vi "initialize.vi"(8 "error in (no error)":errorcluster, 10 "project_file":path, 11 "lv-builder in":refnum<class "lv-builder-default.lvclass">) -> (0 "error out":errorcluster, 3 "lv-builder out":refnum<class "lv-builder-default.lvclass">)   [LabVIEW 2015, in "lv-builder-default.lvclass"]
uses:
  lv-builder-default.lvclass
  <userlib>/antonio-alexander/lv-bin/lv-bin/public/api/v1/advanced/add_data_path_single.vi
  lv-builder/public/accessors/project_file_write.vi
  lv-builder/public/accessors/commit_hash_write.vi
  lv-builder-default.lvlib
  <userlib>/antonio-alexander/lv-bin-git/public/api/v1/v1.lvlib
  <userlib>/antonio-alexander/lv-bin/lv-bin/public/api/v1/v1.lvlib
  <userlib>/antonio-alexander/lv-bin-7zip/lv-bin-7zip.lvlib
  <userlib>/antonio-alexander/lv-bin-git/lv-bin-git.lvlib
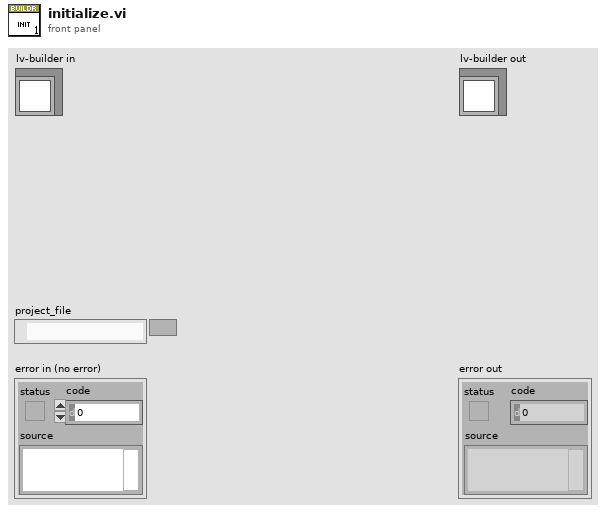
[diagram p1: front panel]
types:
  T1 = typedef "lv-builder-default.lvlib/configuration.ctl" = cluster{"project_file":string, "lvlibp_directory":string, "zip_directory":string, "lvlib_directory":string, "update_version_vi":string, "installer_post_file":string, "distribution_folder":string, "dependencies_folder":string, "version":string, "bin_folder":string, "lvlib_post_action":u16, "installer_post_action":u16, "application_post_action":u16, "zip_post_action":u16}
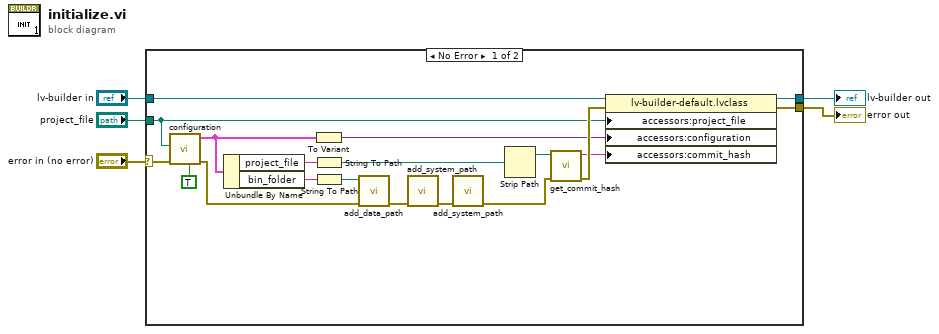
[diagram p0: block diagram]
diagram:
  n1 = case shown="No Error" "error in (no error)" {
    selector: "error in (no error)" -> [w11 w26]
    tunnel: [w22 w26] -> w4
    tunnel: [w23 w25] -> w2
    tunnel: "lv-builder in" -> [w10 w25]
    tunnel: "project_file" -> [w6 _]
    frame No Error {
      n2 = call "configuration.vi"("force_read?"=TRUE, "error in (no error)"=w11, "project_file"=w6) -> ("error out"=w17:errorcluster, "config out"=w21:T1)  [unwired: 7 in]
      n3 = Unbundle By Name(w21) -> ("project_file"=w14:string, "bin_folder"=w8:string)
      n4 = To Variant(anything=w21) -> (Variant=w7:variant)
      n5 = String To Path(string=w14) -> (path=w13:path)
      n6 = String To Path(string=w8) -> (path=w18:path)
      n7 = call-poly <userlib>:"add_data_path.vi"("error in (no error)"=w17, "path_to_add"=w18) -> ("error out"=w20:errorcluster)  [unwired: 9 in]
      n8 = call <userlib>:"add_system_path.vi"("error in (no error)"=w20) -> ("error out"=w19:errorcluster)  [unwired: 10 in]
      n9 = call <userlib>:"add_system_path.vi"("error in (no error)"=w19) -> ("error out"=w15:errorcluster)  [unwired: 10 in]
      n10 = Strip Path(path=w13) -> (stripped path=w12:path)  [unwired: 1 out]
      n11 = call <userlib>:"get_commit_hash.vi"("error in (no error)"=w15, "path"=w12) -> ("error out"=w24:errorcluster, "commit_hash"=w9:string)  [unwired: 8 in]
      n12 = property class="lv-builder-default.lvclass"(reference=w10, error in=w24, "accessors:project_file"=w6, "accessors:configuration"=w7, "accessors:commit_hash"=w9) -> (reference out=w23:refnum<class "lv-builder-default.lvclass">, error out=w22:errorcluster)
    }
    frame Error {
    }
  }
  "error out" <- w4
  "lv-builder out" <- w2
